vi "Actor.vi"(11 "Class":refnum<class "DAQmx - Analog Input Single Sample.lvclass">) -> ()   [LabVIEW 2021, in "DAQmx - Analog Input Single Sample.lvclass"]
uses:
  DAQmx - Analog Input Single Sample.lvclass
  C:/TSA/DAQmx-Bus/Source/DAQmx-Bus.lvclass
  DAQmx-Bus.lvclass/DAQmx-Bus.ctl
  DAQmx - Analog Input Single Sample.lvclass/DAQmx - Analog Input Single Sample.ctl
  <vilib>/Platform/TimedLoop/XDataNode/timing_clust.ctl
  <vilib>/Platform/TimedLoop/XDataNode/nitl_modes.ctl
  <vilib>/Platform/TimedLoop/XDataNode/wakeup.ctl
  <vilib>/DAQmx/read.llb/DAQmx Read (Analog 1D DBL NChan 1Samp).vi
  Properties/Read DAQmx Task.vi
  Properties/Read Update Rate.vi
  Properties/Read timeout.vi
  Properties/Read Values DVR.vi
  Properties/Read Stop.vi
  Properties/Read Sync.vi
  <vilib>/DAQmx/miscellaneous.llb/DAQmx Fill In Error Info.vi
  <vilib>/platform/TimedLoop/XDataNode/XDataNode.xnode
  <resource>/objmgr/daqmx.rc
  <vilib>/Platform/TimedLoop/XDataNode/XDNodeRunTimeDep.lvlib
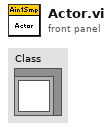
[diagram p1: front panel]
types:
  T1 = typedef "XDNodeRunTimeDep.lvlib/timing_clust.ctl" = cluster{"Expected End [f-1]":u64, "Actual End [f-1]":u64, "Finished Late? [f-1]":bool, "Expected End [i-1]":u64, "Actual End [i-1]":u64, "Finished Late? [i-1]":bool, "Expected Start [i]":u64, "Actual Start [i]":u64, "Expected Start [f]":u64, "Actual Start [f]":u64, "Source Name":string, "Structure Name":string, "Period":i64, "Deadline":i64, "Offset":i64, "Start":i64, "Priority":i32, "Timeout":i32, "Mode":T2, "Wakeup Reason":T3, "Error":errorcluster, "Source Type":string, "Secondary Source Type":string, "Global End Time":u64, "Global Start Time":u64, "Frame Duration":u64, "Iteration Duration":u64, "Assigned CPU":i32, "I/O Scan Engine Mode":u32}
  T2 = typedef "XDNodeRunTimeDep.lvlib/nitl_modes.ctl" = enum32{"No Change", "Process missed periods, maintain original phase", "Discard missed periods, maintain original phase", "Process missed periods, ignore original phase", "Discard missed periods, ignore original phase"}
  T3 = typedef "XDNodeRunTimeDep.lvlib/wakeup.ctl" = enum32{"Normal", "Aborted", "Asynchronous wakeup", "Timing source error", "Timed loop error", "Timeout"}
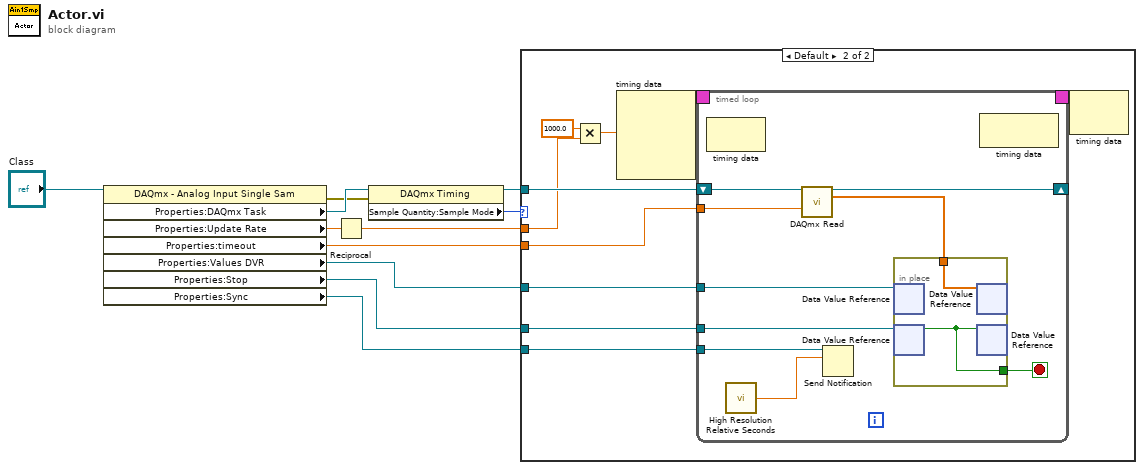
[diagram p0: block diagram]
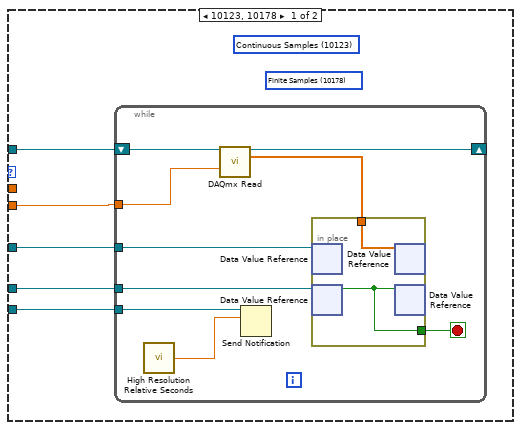
[diagram p2: hidden frame]
diagram:
  n1 = property class="DAQmx - Analog Input Single Sam"(reference="Class") -> (error out=w6:errorcluster, "Properties:DAQmx Task"=w7:refnum<k21>, "Properties:Update Rate"=w3:dbl, "Properties:timeout"=w10:dbl, "Properties:Values DVR"=w9:refnum<data-value>, "Properties:Stop"=w11:refnum<data-value>, "Properties:Sync"=w8:refnum<notifier>)  [unwired: 1 in, 1 out]
  n2 = Reciprocal(x=w3) -> (1/x=w2:dbl)
  n3 = property class="DAQmx Timing"(reference=w7, error in=w6) -> (reference out=w5:refnum<k21>, "Sample Quantity:Sample Mode"=w4:i32)  [unwired: 1 out]
  n4 = case shown="Default" w4 {
    tunnel: w11 -> [w16 w37]
    tunnel: w10 -> [w12 w36]
    tunnel: w9 -> [w15 w35]
    tunnel: w8 -> [w14 w34]
    tunnel: w5 -> [w13 w33]
    tunnel: w2 -> [_ w30]
    frame 10123, 10178 {
      (unwired) 10178 items=["Finite Samples"=10178, "Continuous Samples"=10123, "Hardware Timed Single Point"=12522] ("SampQuant.SampMode")
      (unwired) 10123 items=["Finite Samples"=10178, "Continuous Samples"=10123, "Hardware Timed Single Point"=12522] ("SampQuant.SampMode")
      n5 = while {
        shift-right: [w24] -> _
        shift-left: w13 -> [w25]
        tunnel: w16 -> [w23]
        tunnel: w12 -> [w21]
        tunnel: w15 -> [w20]
        tunnel: w14 -> [w17]
        stop <- w22 stop-if-true
        n6 = call <vilib>:"High Resolution Relative Seconds.vi"() -> ("relative seconds"=w18:dbl)
        n7 = call-poly <vilib>:"DAQmx Read.vi"("task/channels in"=w25, "timeout"=w21) -> ("task out"=w24:refnum<k21>, "data"=w19:dbl[])  [unwired: 11 in, 1 out]
        n8 = Send Notification(notification=w18, notifier=w17) -> ()  [unwired: 1 in, 2 out]
        n9 = in-place {
          in-place-border: [w27] -> w22
          in-place-border: w19 -> [w26]
          n10 = in-place-dvr #1(w20) -> ()  [unwired: 2 out]
          n11 = in-place-dvr #2(w23) -> (w27:bool)  [unwired: 1 out]
          n12 = in-place-dvr #1(w26) -> ()  [unwired: 2 out]
          n13 = in-place-dvr #2(w27) -> ()  [unwired: 2 out]
        }
      }
    }
    frame Default {
      n14 = Multiply(x=1000.0, y=w30) -> (x*y=w28:dbl)
      n15 = node-c288(w28) -> (w32:T1)  [unwired: 3 in]
      n16 = timed-loop {
        shift-right: [w45] -> _
        shift-left: w33 -> [w46]
        tunnel: w37 -> [w44]
        tunnel: w36 -> [w42]
        tunnel: w35 -> [w41]
        tunnel: w34 -> [w38]
        timing: w32 -> [_]
        timing-out: [_] -> w31
        stop <- w43 stop-if-true
        n17 = node-c288() -> ()  [unwired: 1 in, 1 out]
        n18 = call <vilib>:"High Resolution Relative Seconds.vi"() -> ("relative seconds"=w39:dbl)
        n19 = call-poly <vilib>:"DAQmx Read.vi"("task/channels in"=w46, "timeout"=w42) -> ("task out"=w45:refnum<k21>, "data"=w40:dbl[])  [unwired: 11 in, 1 out]
        n20 = Send Notification(notification=w39, notifier=w38) -> ()  [unwired: 1 in, 2 out]
        n21 = in-place {
          in-place-border: [w50] -> w43
          in-place-border: w40 -> [w49]
          n22 = in-place-dvr #3(w41) -> ()  [unwired: 2 out]
          n23 = in-place-dvr #4(w44) -> (w50:bool)  [unwired: 1 out]
          n24 = in-place-dvr #3(w49) -> ()  [unwired: 2 out]
          n25 = in-place-dvr #4(w50) -> ()  [unwired: 2 out]
        }
        n26 = node-c288() -> ()  [unwired: 1 in, 1 out]
      }
      n27 = node-c288(w31) -> ()  [unwired: 1 out]
    }
  }
